vi "FINAL.vi"() -> ()   [LabVIEW 2015]
panel:
  in  "Tab Control":T1(tab)
  in  "PROBABILITY INPUT":dbl[](array[numeric])
  out "SORTED PROBABILITY":dbl[](array[numeric])
  out "INPUT PROBABILITY":dbl[](array[numeric])
  out "CODEWORD 1":dbl[](array[numeric])
  out "CODEWORD 2":dbl[](array[numeric])
  out "CODEWORD  3":dbl[](array[numeric])
  out "CODEWORD  4":dbl[](array[numeric])
  out "LENGTH OF CODE WORD":cluster{sgl, dbl, dbl, dbl}
  out "CODEWORD  1":dbl[](array[numeric])
  out "CODEWORD  2":dbl[](array[numeric])
  out "CODEWORD  3":dbl[](array[numeric])
  out "CODEWORD  4":dbl[](array[numeric])
  out "EFFICIENCY":dbl(knob) scale=0.0..100.0
  out "AVERAGE CODEWORD\n LENGTH":dbl(knob) scale=0.0..5.0
  out "ENTROPY":dbl(knob) scale=0.0..4.0
  out "ENTROPY  2":dbl
  out "ENTROPY":dbl(knob) scale=0.0..4.0
  out "EFFICIENCY  2":dbl
  out "EFFICIENCY":dbl(knob) scale=0.0..100.0
  out "AVG CODE WORD LENGTH":dbl
  out "AVG CODEWORD LENGTH(L)":dbl(knob) scale=0.0..5.0
  out "ENTROPY":dbl
  out "AVERAGE CODEWORD \nLENGTH":dbl
  out "EFFICIENCY 2":dbl
  in  "?":dbl[](array[numeric])
  out "?":i32[][](array[numeric]) format="%b"
  out "?":i32[][](array[numeric])
  # "SHANNON INPUT"
  # "HUFFMAN INPUT"
  # "SHANNON CODE"
  # "HUFFMAN CODE"
  # "SHANNON OUTPUT"
  # "HUFFMAN OUTPUT"
  # "RUNLENGTH"
  # "OUTPUT IN BINARY"
  # "OUTPUT IN DECIMAL"
  # "INPUT"
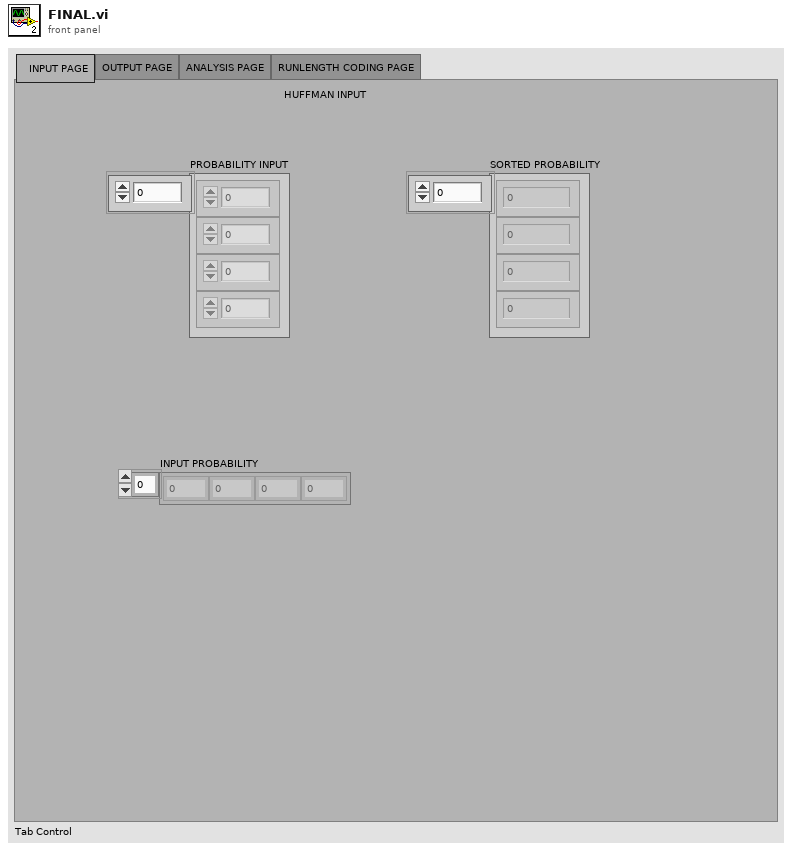
[diagram p1: front panel]
types:
  T1 = enum32{"  INPUT PAGE", "OUTPUT PAGE", "ANALYSIS PAGE", "RUNLENGTH CODING PAGE"}
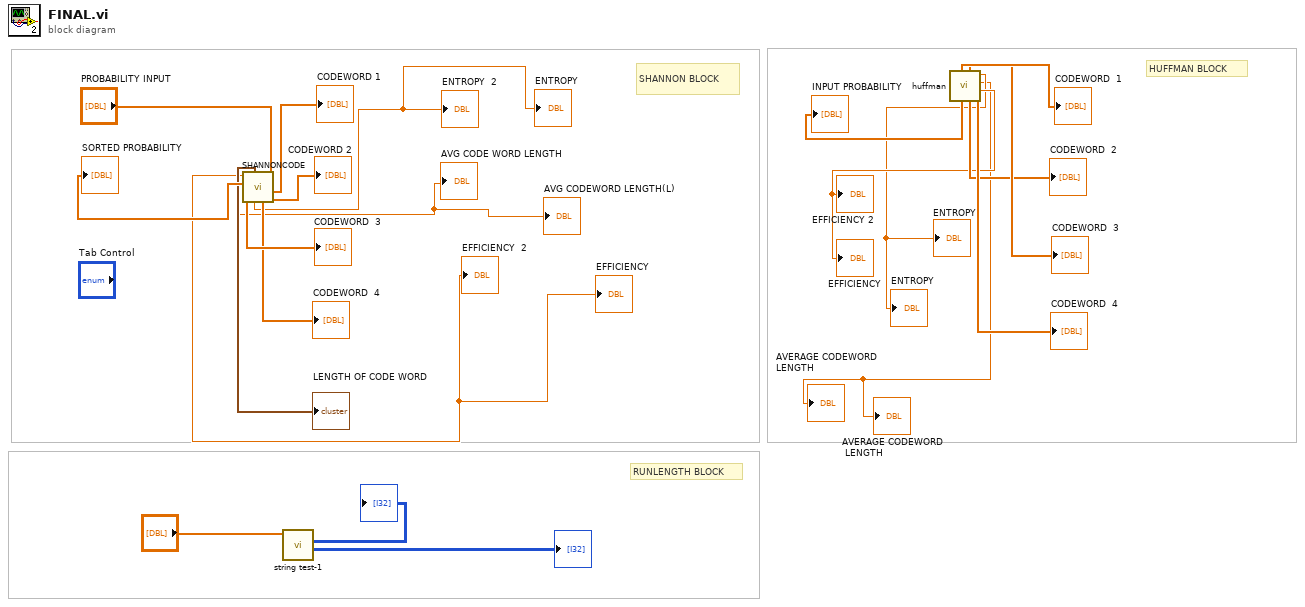
[diagram p0: block diagram]
diagram:
  # "RUNLENGTH BLOCK"
  # "HUFFMAN BLOCK"
  # "SHANNON BLOCK"
  n1 = call "SHANNONCODE.VI"("PROBABILITY INPUT"="PROBABILITY INPUT") -> ("CODEWORD 2"=→"CODEWORD 2":dbl[], "CODEWORD 1"=→"CODEWORD 1":dbl[], "SORTED PROBABILITY"=→"SORTED PROBABILITY":dbl[], "CODEWORD  4"=→"CODEWORD  4":dbl[], "ENTROPY"=→"ENTROPY" →"ENTROPY  2":dbl, "LENGTH OF CODE WORD"=→"LENGTH OF CODE WORD":cluster{sgl, dbl, dbl, dbl}, "CODEWORD  3"=→"CODEWORD  3":dbl[], "AVG CODE WORD LENGTH"=→"AVG CODEWORD LENGTH(L)" →"AVG CODE WORD LENGTH":dbl, "EFFICIENCY"=→"EFFICIENCY" →"EFFICIENCY  2":dbl)  [unwired: 2 in]
  n2 = call "string test-1.vi"("Input"="?") -> ("Output in binary"=→"?":i32[][], "Output in Desimal"=→"?":i32[][])  [unwired: 9 in]
  n3 = call "huffman.vi"() -> ("CODEWORD 4"=→"CODEWORD  4":dbl[], "EFFICIENCY 2"=→"EFFICIENCY 2" →"EFFICIENCY":dbl, "AVERAGE CODEWORD \nLENGTH"=→"AVERAGE CODEWORD \nLENGTH" →"AVERAGE CODEWORD\n LENGTH":dbl, "ENTROPY"=→"ENTROPY" →"ENTROPY":dbl, "CODEWORD 2"=→"CODEWORD  2":dbl[], "CODEWORD 3"=→"CODEWORD  3":dbl[], "INPUT PROBABILITY"=→"INPUT PROBABILITY":dbl[], "CODEWORD 1"=→"CODEWORD  1":dbl[])  [unwired: 4 in]
